vi "Periodic Tasks.vi"(8 "error in":errorcluster) -> ()   [LabVIEW 2016]
doc: "This VI runs in parallel to other tasks. It can contain as many user-defined periodic loops as you need. These can carry out PID or other sorts of timed response."
uses:
  <vilib>/Rock Robotics/Network Tables/NT Read Number.vi
  Robot Global Data.vi
  <vilib>/Rock Robotics/WPI/Solenoid/WPI_SolenoidValue.ctl
  <vilib>/Rock Robotics/WPI/Solenoid/WPI_SolenoidSetEnum.vi
  <vilib>/Rock Robotics/Network Tables/NT Write Number.vi
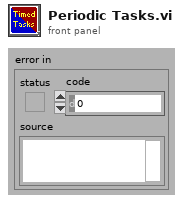
[diagram p1: front panel]
types:
  T1 = typedef "WPI_SolenoidValue.ctl" = enum16{"Off", "On", "Forward", "Reverse"}
  T2 = typedef "WPI_SolenoidDevRef.ctl" = cluster{"DevStatus":errorcluster, "Pneumatics Control Module":u8, "Forward Solenoid Channel":T3, "Reverse Solenoid Channel":T3}
  T3 = typedef "WPI_SolenoidChannel.ctl" = enum8{"Solenoid 0", "Solenoid 1", "Solenoid 2", "Solenoid 3", "Solenoid 4", "Solenoid 5", "Solenoid 6", "Solenoid 7", "Invalid"}
  T4 = typedef "WPI_ServoDeviceRef.ctl" = cluster{"DeviceStatus":errorcluster, "PWM Channel":T5, "DeadBand":T6}
  T5 = typedef "FPGA_DIOPWMChannel.ctl" = enum8{"PWM 0", "PWM 1", "PWM 2", "PWM 3", "PWM 4", "PWM 5", "PWM 6", "PWM 7", "PWM 8", "PWM 9", "PWM MXP 0", "PWM MXP 1", "PWM MXP 2", "PWM MXP 3", "PWM MXP 4", "PWM MXP 5", "PWM MXP 6", "PWM MXP 7", "PWM MXP 8", "PWM MXP 9", "Invalid"}
  T6 = typedef "WPI_PWMDeadband.ctl" = cluster{"Name":string, "maxPositivePwm":i32, "minPositivePwm":i32, "centerPwm":i32, "maxNegativePwm":i32, "minNegativePwm":i32, "angularRange":u16}
  T7 = typedef "WPI_MotorControlDeviceRef.ctl" = cluster{"DeviceStatus":errorcluster, "Type":T8, "PWM":cluster{"PWM Channel":T5, "DeadBand":T6}, "CAN":cluster{"Device Number":u8, "SetOutput VI Ref":variant, "GetOutput VI Ref":variant, "Enable VI Ref":variant, "Disable VI Ref":variant, "Data":variant}, "Invert":bool}
  T8 = typedef "WPI_MotorControlType.ctl" = enum16{"PWM", "CAN"}
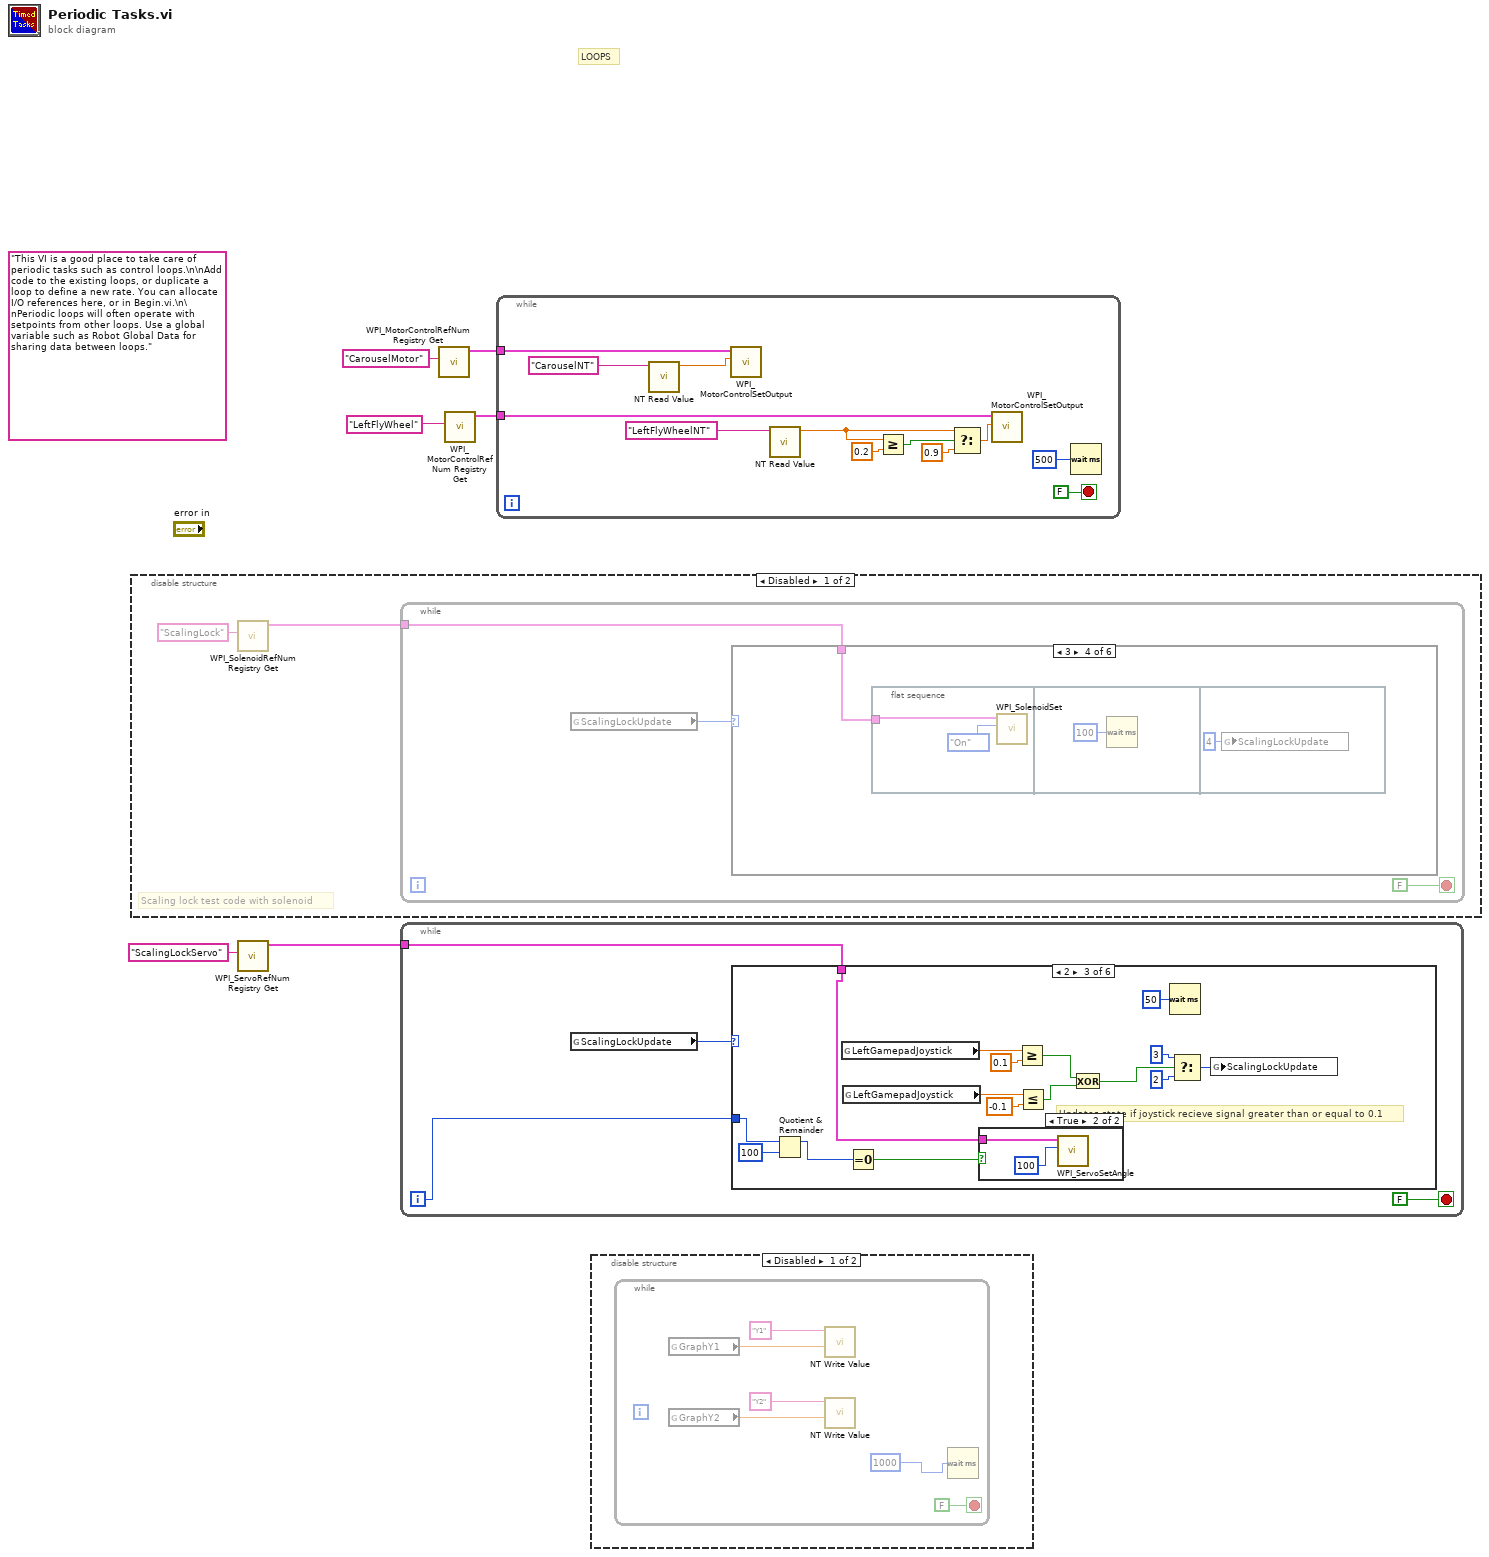
[diagram p0: block diagram]
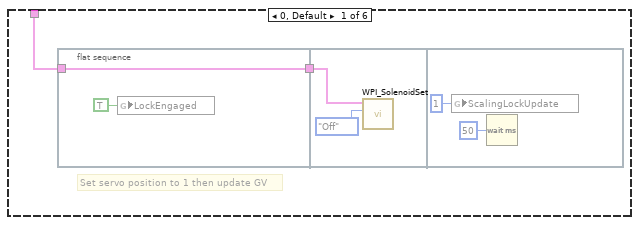
[diagram p2: hidden frame]
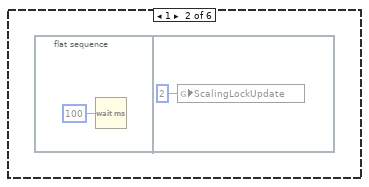
[diagram p3: hidden frame]
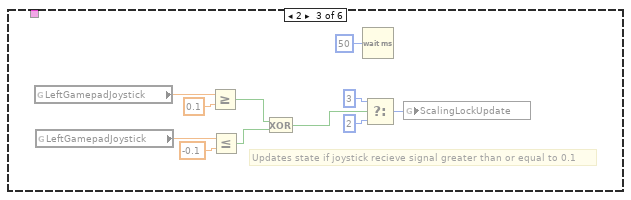
[diagram p4: hidden frame]
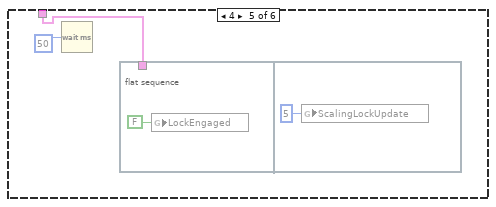
[diagram p5: hidden frame]
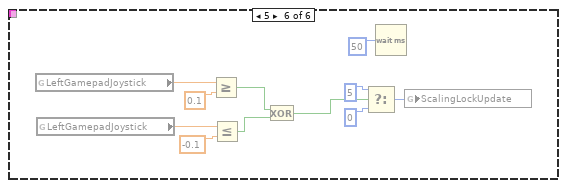
[diagram p6: hidden frame]
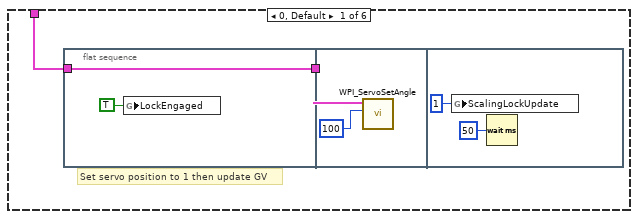
[diagram p9: hidden frame]
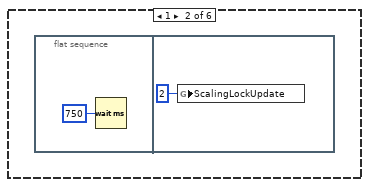
[diagram p10: hidden frame]
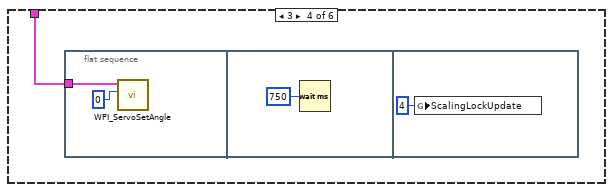
[diagram p12: hidden frame]
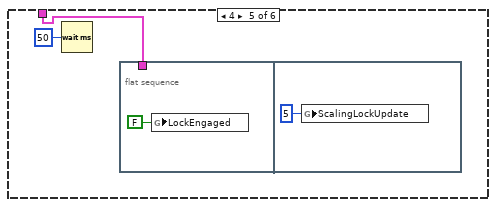
[diagram p13: hidden frame]
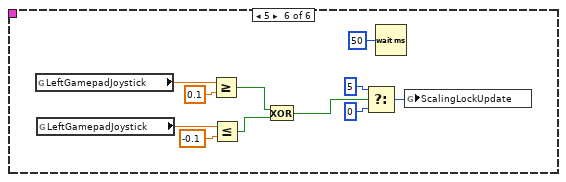
[diagram p14: hidden frame]
diagram:
  (unwired) "This VI is a good place to take care of periodic tasks such as control loops.\n\nAdd code to the existing loops, or duplicate a loop to define a new rate. You can allocate I/O references here, or in Begin.vi.\n\nPeriodic loops will often operate with setpoints from other loops. Use a global variable such as Robot Global Data for sharing data between loops."
  # "LOOPS"
  n1 = disable-structure shown="Disabled" {
    frame Disabled {
      # "Scaling lock test code with solenoid"
      n2 = call <vilib>:"WPI_SolenoidRefNum Registry Get.vi"("refnum name"="ScalingLock") -> ("SolenoidDevRef"=w8:T2)  [unwired: 9 in, 1 out]
      n3 = while {
        tunnel: w8 -> [w9]
        stop <- FALSE stop-if-true
        n4 = global read "Robot Global Data.vi" "ScalingLockUpdate"() -> (w10:i8)
        n5 = case shown="3" w10 {
          tunnel: w9 -> [w13 _ _ w33 w38 _]
          frame 0, Default {
            # "Set servo position to 1 then update GV"
            n6 = flat-sequence {
              tunnel: w13 -> [w15]
              tunnel: [w15] -> w12
              tunnel: w12 -> [w17]
              frame #0 {
                n7 = global write "Robot Global Data.vi" "LockEngaged"(TRUE ("LockEngaged")) -> ()
              }
              frame #1 {
                n8 = call-poly <vilib>:"WPI_SolenoidSet.vi"("Value"=WPI_SolenoidValue."Off", "SolenoidDevRef"=w17) -> ()  [unwired: 8 in, 2 out]
              }
              frame #2 {
                n9 = global write "Robot Global Data.vi" "ScalingLockUpdate"(i8 1 ("ScalingLockUpdate")) -> ()
                n10 = Wait (ms)(milliseconds to wait=u32 50) -> ()  [unwired: 1 out]
              }
            }
          }
          frame 1 {
            n11 = flat-sequence {
              frame #0 {
                n12 = Wait (ms)(milliseconds to wait=u32 100) -> ()  [unwired: 1 out]
              }
              frame #1 {
                n13 = global write "Robot Global Data.vi" "ScalingLockUpdate"(i8 2 ("ScalingLockUpdate")) -> ()
              }
            }
          }
          frame 2 {
            # "Updates state if joystick recieve signal greater than or equal to 0.1"
            n14 = global read "Robot Global Data.vi" "LeftGamepadJoystick"() -> (w32:dbl)
            n15 = global read "Robot Global Data.vi" "LeftGamepadJoystick"() -> (w26:dbl)
            n16 = Greater Or Equal?(x=w32, y=0.1) -> (x >= y?=w24:bool)
            n17 = Less Or Equal?(x=w26, y=-0.1) -> (x <= y?=w23:bool)
            n18 = Exclusive Or(1:w23, 2:w24) -> (0:w22:bool)
            n19 = Wait (ms)(milliseconds to wait=u32 50) -> ()  [unwired: 1 out]
            n20 = Select(t=i8 3, s=w22, f=i8 2) -> (s? t:f=w30:i8)
            n21 = global write "Robot Global Data.vi" "ScalingLockUpdate"(w30) -> ()
          }
          frame 3 {
            n22 = flat-sequence {
              tunnel: w33 -> [w34]
              frame #0 {
                n23 = call-poly <vilib>:"WPI_SolenoidSet.vi"("Value"=WPI_SolenoidValue."On", "SolenoidDevRef"=w34) -> ()  [unwired: 8 in, 2 out]
              }
              frame #1 {
                n24 = Wait (ms)(milliseconds to wait=u32 100) -> ()  [unwired: 1 out]
              }
              frame #2 {
                n25 = global write "Robot Global Data.vi" "ScalingLockUpdate"(i8 4 ("ScalingLockUpdate")) -> ()
              }
            }
          }
          frame 4 {
            n26 = Wait (ms)(milliseconds to wait=u32 50) -> ()  [unwired: 1 out]
            n27 = flat-sequence {
              tunnel: w38 -> [_]
              frame #0 {
                n28 = global write "Robot Global Data.vi" "LockEngaged"(FALSE ("LockEngaged")) -> ()
              }
              frame #1 {
                n29 = global write "Robot Global Data.vi" "ScalingLockUpdate"(i8 5 ("ScalingLockUpdate")) -> ()
              }
            }
          }
          frame 5 {
            n30 = global read "Robot Global Data.vi" "LeftGamepadJoystick"() -> (w52:dbl)
            n31 = global read "Robot Global Data.vi" "LeftGamepadJoystick"() -> (w47:dbl)
            n32 = Greater Or Equal?(x=w52, y=0.1) -> (x >= y?=w45:bool)
            n33 = Less Or Equal?(x=w47, y=-0.1) -> (x <= y?=w44:bool)
            n34 = Exclusive Or(1:w44, 2:w45) -> (0:w43:bool)
            n35 = Select(t=i8 5, s=w43, f=i8 0) -> (s? t:f=w50:i8)
            n36 = Wait (ms)(milliseconds to wait=u32 50) -> ()  [unwired: 1 out]
            n37 = global write "Robot Global Data.vi" "ScalingLockUpdate"(w50) -> ()
          }
        }
      }
    }
    frame Enabled {
    }
  }
  n38 = call <vilib>:"WPI_ServoRefNum Registry Get.vi"("refnum name"="ScalingLockServo") -> ("ServoDeviceRef"=w2:T4)  [unwired: 9 in, 1 out]
  n39 = while {
    tunnel: w2 -> [w54]
    i -> [w53]
    stop <- FALSE stop-if-true
    n40 = global read "Robot Global Data.vi" "ScalingLockUpdate"() -> (w55:i8)
    n41 = case shown="2" w55 {
      tunnel: w54 -> [w58 _ w71 w85 w90 _]
      tunnel: w53 -> [_ _ w70 _ _ _]
      frame 0, Default {
        # "Set servo position to 1 then update GV"
        n42 = flat-sequence {
          tunnel: w58 -> [w60]
          tunnel: [w60] -> w57
          tunnel: w57 -> [w62]
          frame #0 {
            n43 = global write "Robot Global Data.vi" "LockEngaged"(TRUE ("LockEngaged")) -> ()
          }
          frame #1 {
            n44 = call <vilib>:"WPI_ServoSetAngle.vi"("Angle"=100, "ServoDeviceRef"=w62) -> ()  [unwired: 8 in, 2 out]
          }
          frame #2 {
            n45 = global write "Robot Global Data.vi" "ScalingLockUpdate"(i8 1 ("ScalingLockUpdate")) -> ()
            n46 = Wait (ms)(milliseconds to wait=u32 50) -> ()  [unwired: 1 out]
          }
        }
      }
      frame 1 {
        n47 = flat-sequence {
          frame #0 {
            n48 = Wait (ms)(milliseconds to wait=u32 750) -> ()  [unwired: 1 out]
          }
          frame #1 {
            n49 = global write "Robot Global Data.vi" "ScalingLockUpdate"(i8 2 ("ScalingLockUpdate")) -> ()
          }
        }
      }
      frame 2 {
        # "Updates state if joystick recieve signal greater than or equal to 0.1"
        n50 = Quotient & Remainder(x=w70, y=100) -> (x-y*floor(x/y)=w68:i32)  [unwired: 1 out]
        n51 = global read "Robot Global Data.vi" "LeftGamepadJoystick"() -> (w82:dbl)
        n52 = global read "Robot Global Data.vi" "LeftGamepadJoystick"() -> (w76:dbl)
        n53 = Equal To 0?(x=w68) -> (x = 0?=w67:bool)
        n54 = case shown="True" w67 {
          tunnel: w71 -> [_ w83]
          frame False {
          }
          frame True {
            n55 = call <vilib>:"WPI_ServoSetAngle.vi"("Angle"=100, "ServoDeviceRef"=w83) -> ()  [unwired: 8 in, 2 out]
          }
        }
        n56 = Greater Or Equal?(x=w82, y=0.1) -> (x >= y?=w74:bool)
        n57 = Less Or Equal?(x=w76, y=-0.1) -> (x <= y?=w73:bool)
        n58 = Exclusive Or(1:w73, 2:w74) -> (0:w72:bool)
        n59 = Wait (ms)(milliseconds to wait=u32 50) -> ()  [unwired: 1 out]
        n60 = Select(t=i8 3, s=w72, f=i8 2) -> (s? t:f=w80:i8)
        n61 = global write "Robot Global Data.vi" "ScalingLockUpdate"(w80) -> ()
      }
      frame 3 {
        n62 = flat-sequence {
          tunnel: w85 -> [w86]
          frame #0 {
            n63 = call <vilib>:"WPI_ServoSetAngle.vi"("Angle"=0, "ServoDeviceRef"=w86) -> ()  [unwired: 8 in, 2 out]
          }
          frame #1 {
            n64 = Wait (ms)(milliseconds to wait=u32 750) -> ()  [unwired: 1 out]
          }
          frame #2 {
            n65 = global write "Robot Global Data.vi" "ScalingLockUpdate"(i8 4 ("ScalingLockUpdate")) -> ()
          }
        }
      }
      frame 4 {
        n66 = Wait (ms)(milliseconds to wait=u32 50) -> ()  [unwired: 1 out]
        n67 = flat-sequence {
          tunnel: w90 -> [_]
          frame #0 {
            n68 = global write "Robot Global Data.vi" "LockEngaged"(FALSE ("LockEngaged")) -> ()
          }
          frame #1 {
            n69 = global write "Robot Global Data.vi" "ScalingLockUpdate"(i8 5 ("ScalingLockUpdate")) -> ()
          }
        }
      }
      frame 5 {
        n70 = global read "Robot Global Data.vi" "LeftGamepadJoystick"() -> (w104:dbl)
        n71 = global read "Robot Global Data.vi" "LeftGamepadJoystick"() -> (w99:dbl)
        n72 = Greater Or Equal?(x=w104, y=0.1) -> (x >= y?=w97:bool)
        n73 = Less Or Equal?(x=w99, y=-0.1) -> (x <= y?=w96:bool)
        n74 = Exclusive Or(1:w96, 2:w97) -> (0:w95:bool)
        n75 = Select(t=i8 5, s=w95, f=i8 0) -> (s? t:f=w102:i8)
        n76 = Wait (ms)(milliseconds to wait=u32 50) -> ()  [unwired: 1 out]
        n77 = global write "Robot Global Data.vi" "ScalingLockUpdate"(w102) -> ()
      }
    }
  }
  n78 = call <vilib>:"WPI_MotorControlRefNum Registry Get.vi"("refnum name"="CarouselMotor") -> ("MotorControlDevRef"=w5:T7)  [unwired: 9 in, 1 out]
  n79 = call <vilib>:"WPI_MotorControlRefNum Registry Get.vi"("refnum name"="LeftFlyWheel") -> ("MotorControlDevRef"=w6:T7)  [unwired: 9 in, 1 out]
  n80 = while {
    tunnel: w6 -> [w115]
    tunnel: w5 -> [w113]
    stop <- FALSE stop-if-true
    n81 = call-poly <vilib>:"NT Read Value.vi"("Name"="CarouselNT") -> ("Numeric"=w112:dbl)  [unwired: 9 in, 1 out]
    n82 = call <vilib>:"WPI_MotorControlSetOutput.vi"("Output"=w112, "MotorControlDevRef"=w113) -> ()  [unwired: 7 in, 3 out]
    n83 = call-poly <vilib>:"NT Read Value.vi"("Name"="LeftFlyWheelNT") -> ("Numeric"=w106:dbl)  [unwired: 9 in, 1 out]
    n84 = Greater Or Equal?(x=w106, y=0.2) -> (x >= y?=w108:bool)
    n85 = Select(t=w106, s=w108, f=0.9) -> (s? t:f=w105:dbl)
    n86 = call <vilib>:"WPI_MotorControlSetOutput.vi"("Output"=w105, "MotorControlDevRef"=w115) -> ()  [unwired: 7 in, 3 out]
    n87 = Wait (ms)(milliseconds to wait=u32 500) -> ()  [unwired: 1 out]
  }
  n88 = disable-structure shown="Disabled" {
    frame Disabled {
      n89 = while {
        stop <- FALSE stop-if-true
        n90 = global read "Robot Global Data.vi" "GraphY1"() -> (w120:dbl)
        n91 = global read "Robot Global Data.vi" "GraphY2"() -> (w119:dbl)
        n92 = call-poly <vilib>:"NT Write Value.vi"("Numeric"=w120, "Name"="Y1") -> ()  [unwired: 9 in, 1 out]
        n93 = call-poly <vilib>:"NT Write Value.vi"("Numeric"=w119, "Name"="Y2") -> ()  [unwired: 9 in, 1 out]
        n94 = Wait (ms)(milliseconds to wait=u32 1000) -> ()  [unwired: 1 out]
      }
    }
    frame Enabled {
    }
  }
